vi "CSM Reuse Module.vi"(5 "Init State (\"Macro: Initialize\")":string="Macro: Initialize", 7 "Name (\"\" to Use UUID)":string="Reuse Module") -> ()   [LabVIEW 2017, in "1. Create a reuse Module.lvlib"]
doc: "#### Overview\n\nIn the CSM framework, creating a reusable module usually does not require message interaction with other modules. You only need to provide external interfaces and publish the module's state changes. Therefore, as long as these two aspects are clearly described, the reusable module can be called even without knowledge of its internal implementation details. This example demonstrates how to create a reusable module that checks if random data exceeds a user-defined threshold.\n\nIn a CSM module, all case branches can be considered callable messages, but it is recommended to use API groups as external interfaces. When state updates need to be sent, Status or Interrupt Status can be sent to notify external modules of internal state changes.\n\n#### Introduction\n\nThis example demonstrates a CSM module whose function is to generate a random number every second and compare that number with a user-defined threshold. When the generated random number exceeds the threshold, an update is broadcast.\n\n#### Steps\n\n- Step1: Drag and drop the CSM Template from the palette.\n- Step2: Add <b>Level</b> to Internal Data. The default value is 0.5.\n- Step3: Create \"DoSth: Check If Greater than 0.5\" to implement the core functionality.\n - Step3.1: Compare random data and update the UI.\n - Step3.2: Publish the \"Status Changed\" status when random data exceeds the level.\n- Step4: Change the <b>Timeout</b> to a shift register. It will be used to start/stop timeout events. Wire <b>Timeout</b> in every case.\n- Step5: In the Timeout Event, add \"DoSth: Check If Greater than 0.5\" to the State Queue.\n- Step6: Create APIs for this module.\n - Step6.1: Create \"API: Start\" to change the timeout to 0.5, which will trigger \"DoSth: Check If Greater than 0.5\" every second. In this case, broadcast the \"Check Started\" status.\n - Step6.2: Create \"API: Stop\" to change the timeout to -1, which will stop the checking. The \"Check Stopped\" status will be broadcast.\n - Step6.3: Create \"API: Set Level\" to change the Level setting.\n - Step6.4: Create \"API: Get Level\" to retrieve the current Level from the outside.\n- Step7: Create local test buttons/controls.\n - Step7.1: Create a <b>Level</b> control and call \"API: Set Level\" to change the level setting locally.\n - Step7.2: Create a <b>Start</b> button and call \"API: Start\" to begin checking locally.\n - Step7.3: Create a <b>Stop</b> button and call \"API: Stop\" to stop checking locally.\n- Step8: Correctly update the UI where appropriate.\n - Step8.1: Initialize the UI at startup.\n - Step8.2: Comment out `UI: Front Panel State >> Open` in \"Macro: Initialize\". When working as a submodule, the UI will automatically hide instead of popping up."
uses:
  1. Create a reuse Module.lvlib
  user.lib/_NEVSTOP/Communicable State Machine(CSM)/AdvanceAPI/CSM - Break Down Multiple States String.vi
  user.lib/_NEVSTOP/Communicable State Machine(CSM)/AdvanceAPI/CSM - Compact Multiple States.vi
  user.lib/_NEVSTOP/Communicable State Machine(CSM)/AdvanceAPI/CSM - Make String Arguments Safe.vi
  user.lib/_NEVSTOP/Communicable State Machine(CSM)/AdvanceAPI/CSM - Keywords.vi
  user.lib/_NEVSTOP/Communicable State Machine(CSM)/Communicable State Machine.lvlib
panel:
  in  "Level":dbl=0.5 min=0.0 max=1.0 step=0.1 format="%#_13g"
  in  "Stop":bool
  in  "Start":bool
  out "publish status":bool
  out "Random":dbl
  out "State History":string
  # "#CSM-Example Overview\n\nIn the CSM framework, creating a reusable module usually does not require message interaction with other modules. You only need to provide external interfaces and publish the module's state changes. Therefore, as long as these two aspects are clearly described, the reusable module can be called even without knowledge of its internal implementation details. This example demonstrates how to create a reusable module that checks if random data exceeds a user-defined threshold.\n\nIn a CSM module, all case branches can be considered callable messages, but it is recommended to use API groups as external interfaces. When state updates need to be sent, Status or Interrupt Status can be sent to notify external modules of internal state changes."
  # "If"
  # ">"
  # ", Then"
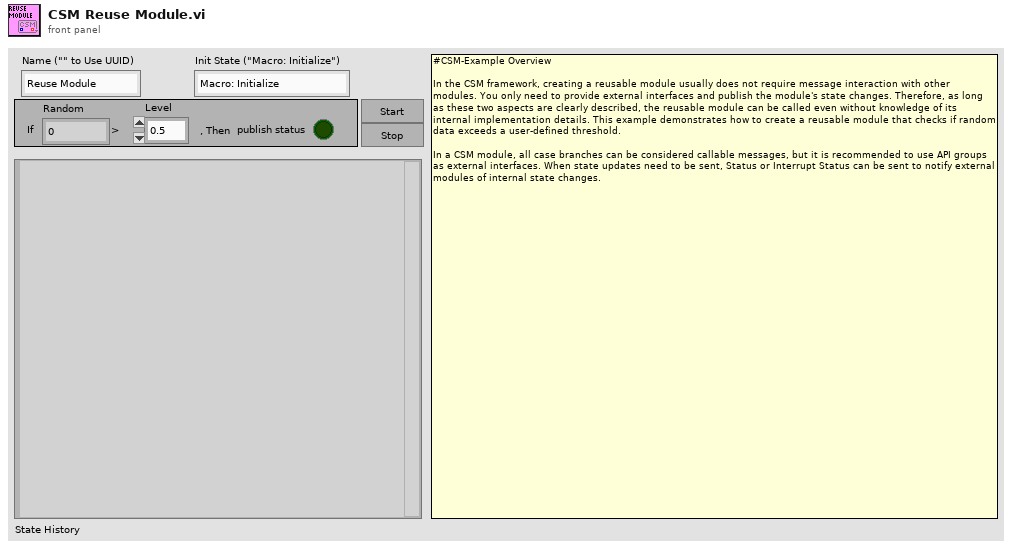
[diagram p1: front panel]
types:
  T1 = enum32{"Invalid", "Standard", "Closed", "Hidden", "Minimized", "Maximized"}
  T2 = enum32{"invalid app kind", "Development System", "Run Time System", "Student Edition", "Embedded LabVIEW", "Evaluation", "Custom"}
  T3 = typedef "Communicable State Machine.lvlib/_CSM_Response Source Message.ctl" = cluster{"‘State":string, "’Arguments":string, "’Error":errorcluster}
  T4 = cluster{"Current VI Reference":refnum<vi>, "Close Panel on Exit?":bool}
  T5 = cluster{"Core":cluster{"Current VI Reference":refnum<vi>, "Close Panel on Exit?":bool}, "Level":dbl}
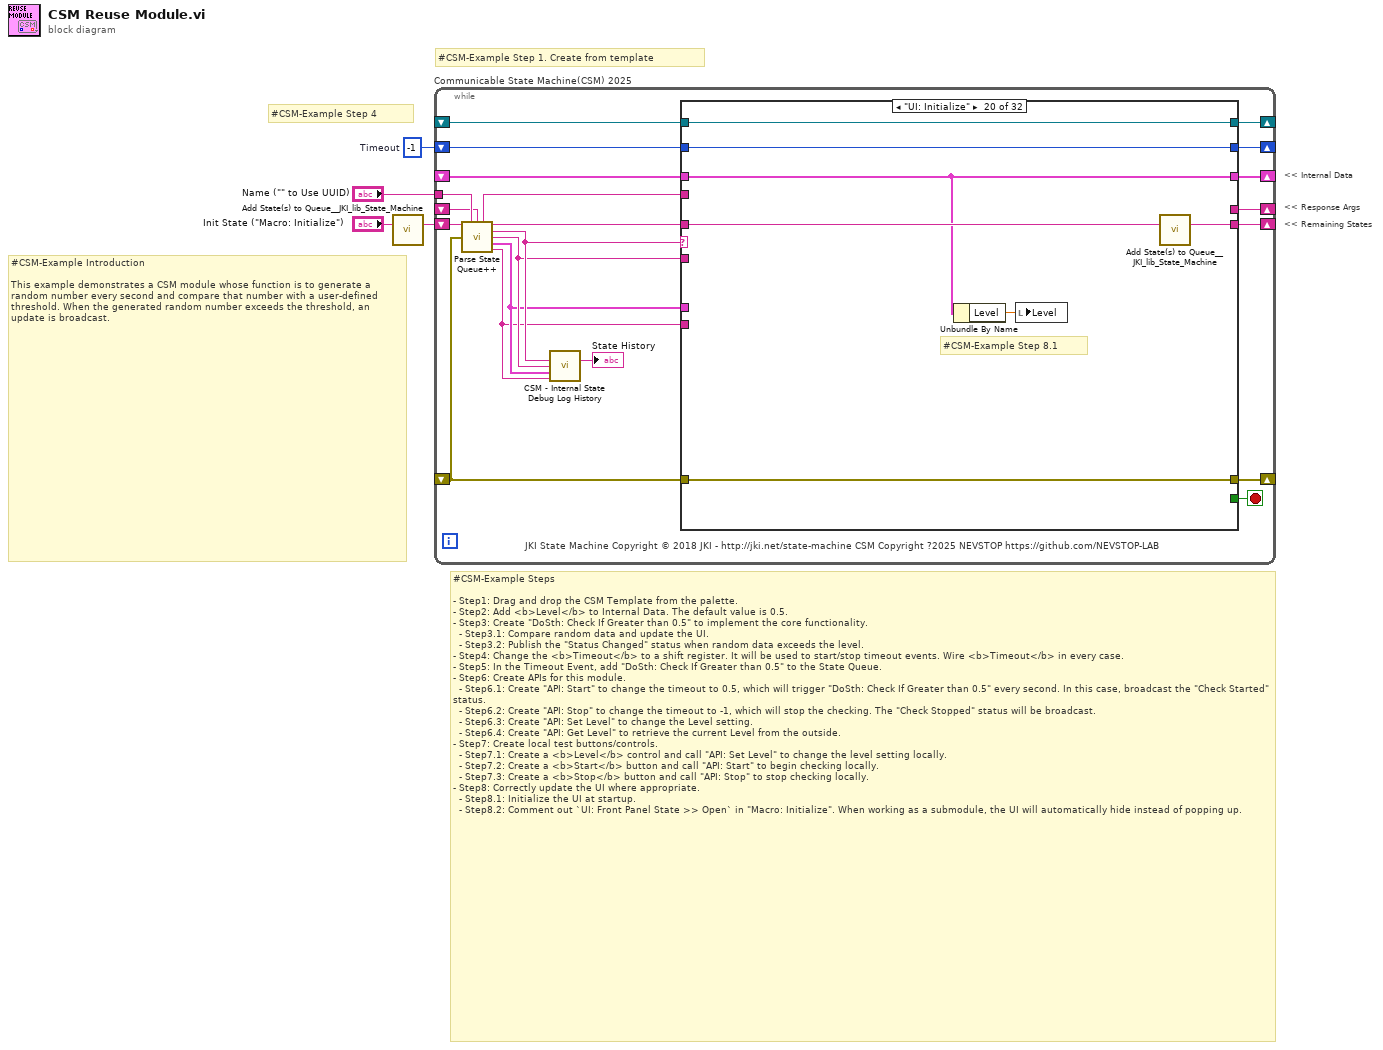
[diagram p0: block diagram]
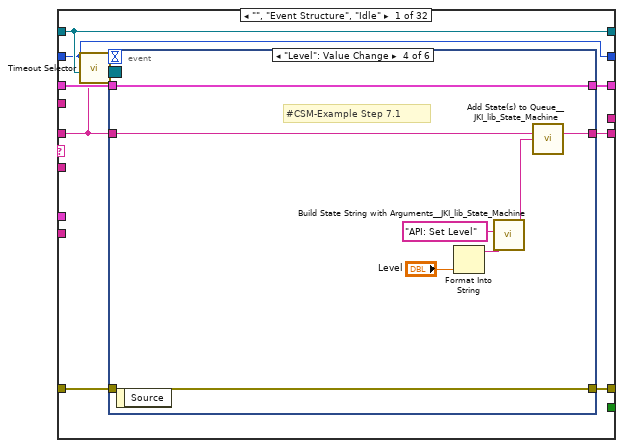
[diagram p2: hidden frame]
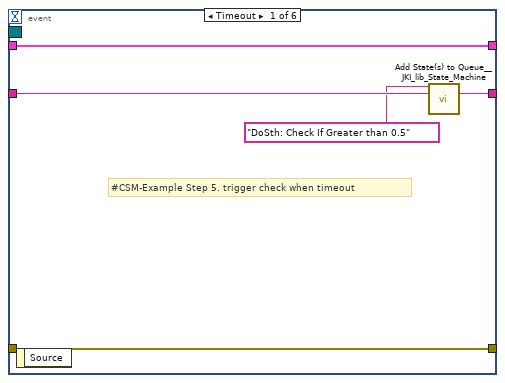
[diagram p3: hidden frame]
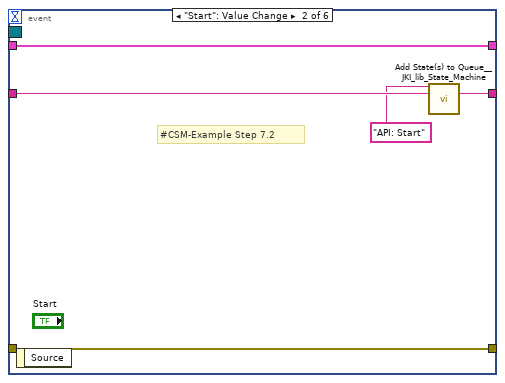
[diagram p4: hidden frame]
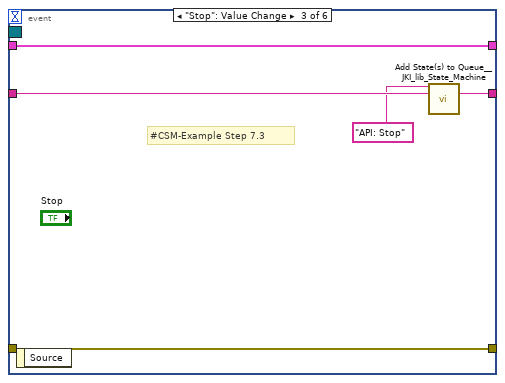
[diagram p5: hidden frame]
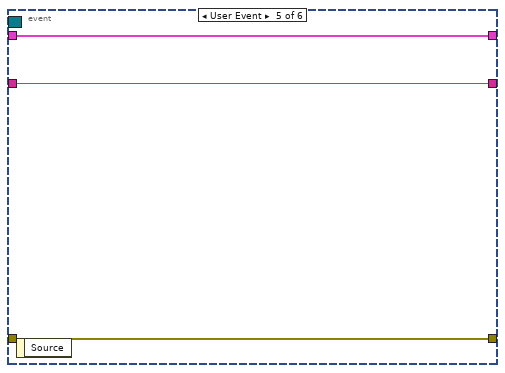
[diagram p6: hidden frame]
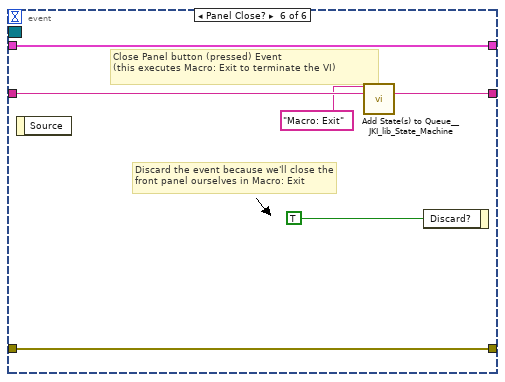
[diagram p7: hidden frame]
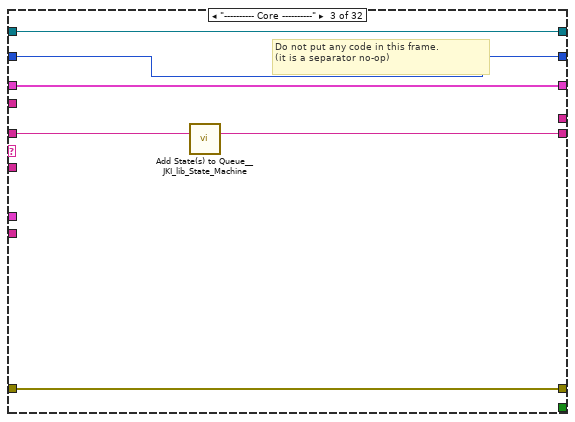
[diagram p9: hidden frame]
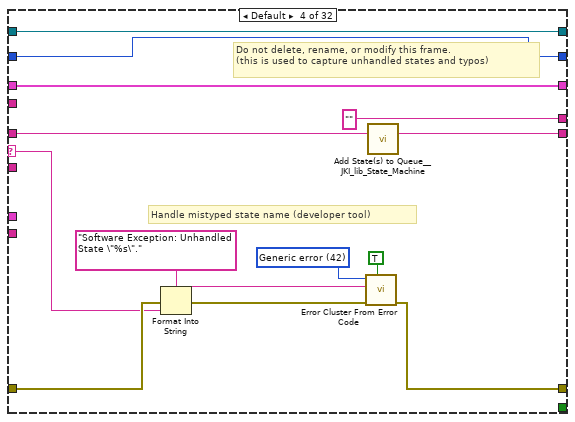
[diagram p10: hidden frame]
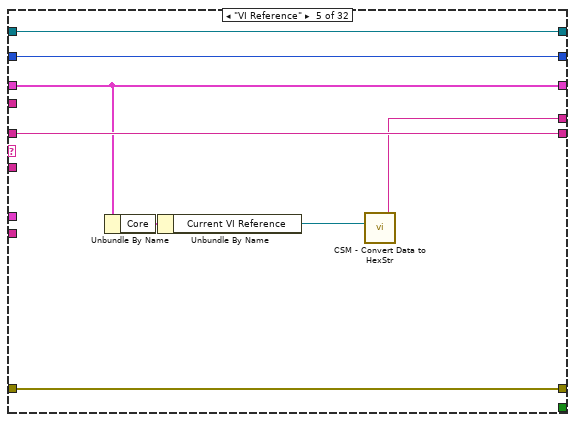
[diagram p11: hidden frame]
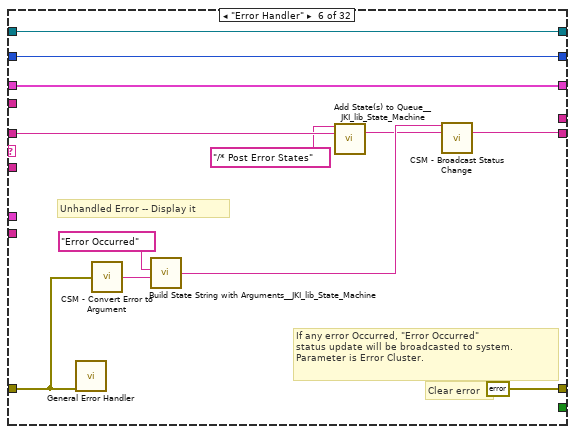
[diagram p12: hidden frame]
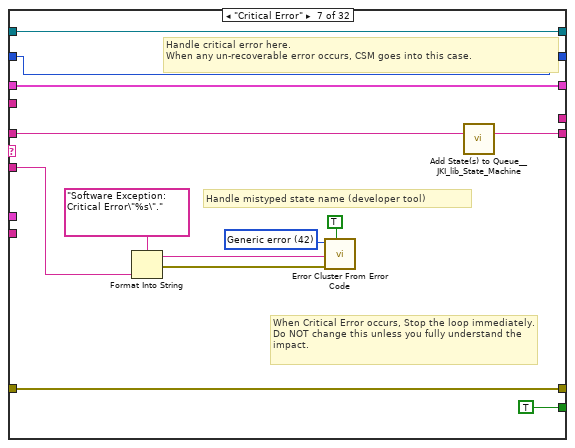
[diagram p13: hidden frame]
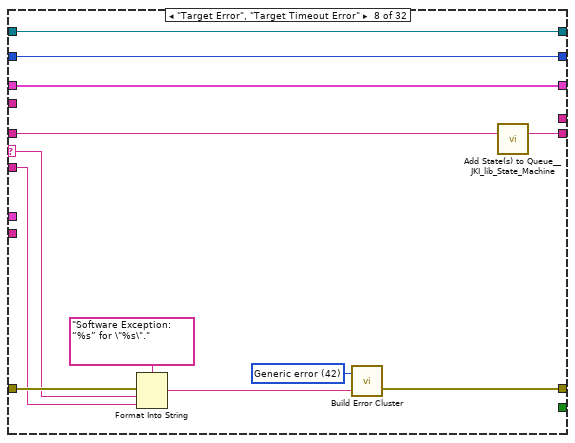
[diagram p14: hidden frame]
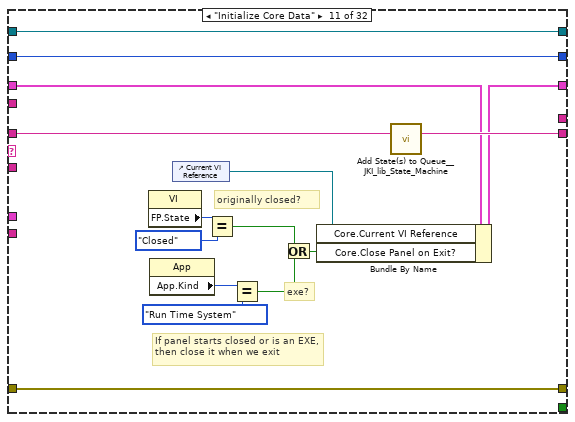
[diagram p17: hidden frame]
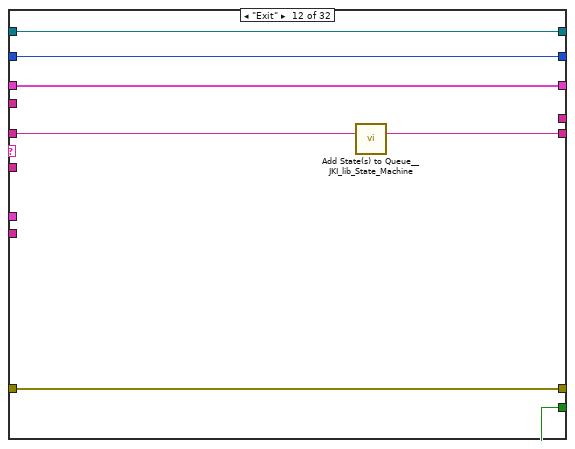
[diagram p18: hidden frame]
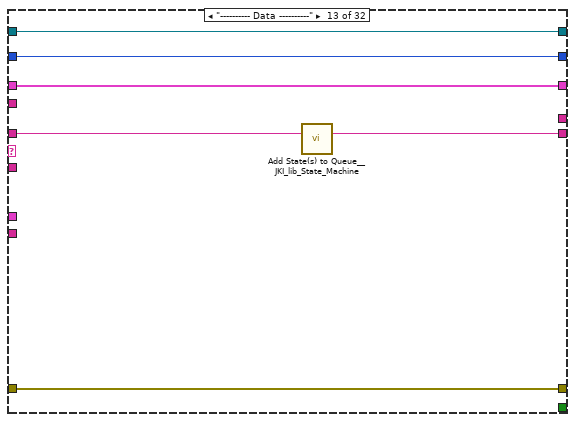
[diagram p19: hidden frame]
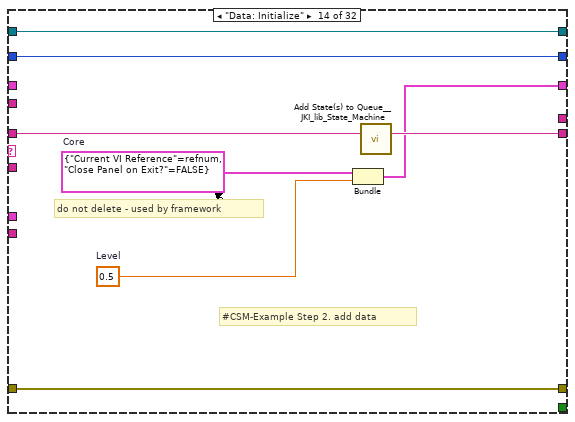
[diagram p20: hidden frame]
diagram:
  w2 = -1  # Timeout
  # "#CSM-Example Introduction\n\nThis example demonstrates a CSM module whose function is to generate a random number every second and compare that number with a user-defined threshold. When the generated random number exceeds the threshold, an update is broadcast."
  # "#CSM-Example Steps\n\n- Step1: Drag and drop the CSM Template from the palette.\n- Step2: Add <b>Level</b> to Internal Data. The default value is 0.5.\n- Step3: Create \"DoSth: Check If Greater than 0.5\" to implement the core functionality.\n  - Step3.1: Compare random data and update the UI.\n  - Step3.2: Publish the \"Status Changed\" status when random data exceeds the level.\n- Step4: Change the <b>Timeout</b> to a shift register. It will be used to start/stop timeout events. Wire <b>Timeout</b> in every case.\n- Step5: In the Timeout Event, add \"DoSth: Check If Greater than 0.5\" to the State Queue.\n- Step6: Create APIs for this module.\n  - Step6.1: Create \"API: Start\" to change the timeout to 0.5, which will trigger \"DoSth: Check If Greater than 0.5\" every second. In this case, broadcast the \"Check Started\" status.\n  - Step6.2: Create \"API: Stop\" to change the timeout to -1, which will stop the checking. The \"Check Stopped\" status will be broadcast.\n  - Step6.3: Create \"API: Set Level\" to change the Level setting.\n  - Step6.4: Create \"API: Get Level\" to retrieve the current Level from the outside.\n- Step7: Create local test buttons/controls.\n  - Step7.1: Create a <b>Level</b> control and call \"API: Set Level\" to change the level setting locally.\n  - Step7.2: Create a <b>Start</b> button and call \"API: Start\" to begin checking locally.\n  - Step7.3: Create a <b>Stop</b> button and call \"API: Stop\" to stop checking locally.\n- Step8: Correctly update the UI where appropriate.\n  - Step8.1: Initialize the UI at startup.\n  - Step8.2: Comment out `UI: Front Panel State >> Open` in \"Macro: Initialize\". When working as a submodule, the UI will automatically hide instead of popping up."
  # "#CSM-Example Step 4"
  # "#CSM-Example Step 1. Create from template"
  # "<< Internal Data"
  # "<< Response Args"
  # "<< Remaining States"
  n1 = call <vilib>:"Add State(s) to Queue__JKI_lib_State_Machine.vi"("State(s) in (\"\")"="Init State (\"Macro: Initialize\")") -> ("States Out"=w4:string)  [unwired: 14 in]
  n2 = while "Communicable State Machine(CSM) 2025" {
    shift-right: [w20] -> _
    shift-left: _ -> [w19]
    shift-right: [w23] -> _
    shift-left: _ -> [w18]
    shift-right: [w22] -> _
    shift-left: w4 -> [w24]
    tunnel: "Name (\"\" to Use UUID)" -> [w14]
    shift-right: [w17] -> _
    shift-left: _ -> [w8]
    shift-right: [w16] -> _
    shift-left: _ -> [w15]
    shift-right: [w6] -> _
    shift-left: w2 -> [w7]
    stop <- w21 stop-if-true
    # "JKI State Machine Copyright © 2018 JKI - http://jki.net/state-machine CSM Copyright ?2025 NEVSTOP https://github.com/NEVSTOP-LAB"
    n3 = call "Parse State Queue++.vi"("State Queue"=w24, "Name (\"\" to Use UUID)"=w14, "Response Arguments"=w8, "Previous Error"=w18) -> ("Name Used"=w9:string, "Remaining States"=w25:string, "Current State"=w13:string, "Arguments"=w12:string, "Additional Information"=w11:T3, "Source CSM"=w10:string)  [unwired: 6 in]
    n4 = call "CSM - Internal State Debug Log History.vi"("State"=w13, "Arguments (\"\")"=w12, ">> Response Source Message >>"=w11, "Source (\"\")"=w10) -> ("Debug Log"=→"State History":string)  [unwired: 11 in]
    n5 = case shown="\"UI: Initialize\"" w13 {
      selector: w13 -> [_ _ _ w81 _ _ _ w126 _ _ _ _ _ _ _ _ _ _ _ _ _ _ _ _ _ _ _ _ _ _ _ _]
      tunnel: w25 -> [w27 w70 w77 w85 w98 w111 w122 w128 w140 w145 w161 w168 w174 w182 w190 w196 w203 w208 w215 w222 w230 w247 w318 w325 w337 w341 w348 w355 w363 w370 w377 w391]
      tunnel: w12 -> [_ _ _ _ _ _ w115 w127 _ _ _ _ _ _ _ _ _ _ _ _ w225 w241 _ _ _ _ _ _ w358 _ _ _]
      tunnel: w19 -> [w33 w69 w74 w83 w97 w109 w123 w130 w139 w144 w154 w166 w171 _ w185 w193 w202 w207 w212 w217 w228 w243 w315 w322 w334 w340 w347 w354 w362 w367 w374 w382]
      tunnel: [w32 w71 w75 w87 w99 errorcluster {"status"=FALSE, "code"=0, "source"=""} ("error out") w124 w133 w141 w146 w158 w165 w172 w179 w186 w194 w198 w206 w213 w220 w226 w244 w316 w323 w335 w342 w349 w356 w364 w371 w375 w389] -> w23
      tunnel: w18 -> [w31 w71 w75 w86 w99 w100 w124 w132 w141 w146 w158 w165 w172 w179 w187 w194 _ w209 w213 w220 w227 w245 w316 w323 w335 w342 w349 w356 w364 w371 w375 w389]
      tunnel: [w34 w70 w76 w84 w98 w102 w121 w131 w140 w145 w160 w167 w173 w181 w189 w195 w203 w208 w214 w221 w229 w246 w317 w324 w336 w341 w344 w351 w363 w370 w376 w390] -> w22
      tunnel: [_ _ _ _ _ _ TRUE _ _ _ _ TRUE _ _ _ _ _ _ _ _ _ _ _ _ _ _ _ _ _ _ _ _] -> w21
      tunnel: [w30 w69 w74 w83 w97 w109 w123 w130 w139 w144 w159 w166 w171 w180 w185 w193 w202 w207 w212 w217 w228 w243 w315 w322 w334 w340 w347 w354 w359 w367 w374 w382] -> w20
      tunnel: w7 -> [w26 w67 w72 w78 w95 w101 w112 w125 w137 w142 w147 w162 w169 w176 w183 w191 w197 w204 w210 w218 w223 w239 w313 w319 w326 w338 _ _ w360 w368 w372 w383]
      tunnel: w10 -> [_ _ _ _ _ _ _ _ _ _ _ _ _ _ _ _ _ _ _ _ _ _ _ _ _ _ _ _ _ _ _ _]
      tunnel: w11 -> [_ _ _ _ _ _ _ _ _ _ _ _ _ _ _ _ _ _ _ _ _ _ _ _ _ _ _ _ _ _ _ _]
      tunnel: [_ _ _ "" w92 _ _ _ _ _ _ _ _ _ _ _ _ _ _ _ _ _ _ _ _ _ _ _ _ w365 _ _] -> w17
      tunnel: [w29 w68 w73 w79 w96 w107 w113 w129 w138 w143 w148 w163 w170 w177 w184 w192 w201 w205 w211 w219 w224 w240 w314 w320 w327 w339 w346 w353 w361 w369 w373 w388] -> w16
      tunnel: w15 -> [w29 w68 w73 w79 w96 w107 w113 w129 w138 w143 w148 w163 w170 w177 w184 w192 _ w205 w211 w219 w224 w240 w314 w320 w327 w339 w346 w353 w361 w369 w373 w388]
      tunnel: w9 -> [_ _ _ _ _ _ _ _ _ _ _ _ _ _ _ _ w200 _ _ _ _ _ _ _ _ _ _ _ _ _ _ _]
      tunnel: [w26 w67 w72 w78 w95 w101 w112 w125 w137 w142 w147 w162 w169 w176 w183 w191 w197 w204 w210 w218 w223 w239 w313 w319 w326 w338 500 ("Timeout") -1 ("Timeout") w360 w368 w372 w383] -> w6
      frame "", "Event Structure", "Idle" {
        n6 = call "Timeout Selector.vi"("Remaining States"=w27, "Timeout Expected"=w26) -> ("Timeout"=w28:i32)  [unwired: 5 in]
        n7 = event shown="[3] \"Level\": Value Change" {
          selector: w29 -> [_ _ _ _ _ _]
          dyn-events: _ -> [_ _ _ _ _ _]
          timeout: w28 -> [_ _ _ _ _ _]
          tunnel: w27 -> [w39 w44 w49 w55 w59 w66]
          tunnel: [w38 w43 w48 w54 w59 w65] -> w34
          tunnel: w33 -> [w36 w41 w46 w56 w60 w63]
          tunnel: [w37 w42 w47 w57 w58 w64] -> w32
          tunnel: w31 -> [w37 w42 w47 w57 w58 w64]
          tunnel: [w36 w41 w46 w56 w60 w63] -> w30
          event Timeout {
            # "#CSM-Example Step 5. trigger check when timeout"
            n8 = event-data() -> ()  [unwired: 1 in, 1 out]
            n9 = call <vilib>:"Add State(s) to Queue__JKI_lib_State_Machine.vi"("State(s) in Front (\"\")"="DoSth: Check If Greater than 0.5" ("State(s) in Front (\"\")"), "State(s) in (\"\")"=w39) -> ("States Out"=w38:string)  [unwired: 13 in]
          }
          event "Start": Value Change {
            # "#CSM-Example Step 7.2"
            n10 = event-data() -> ()  [unwired: 1 in, 1 out]
            n11 = call <vilib>:"Add State(s) to Queue__JKI_lib_State_Machine.vi"("State(s) in Front (\"\")"="API: Start" ("State(s) in Front (\"\")"), "State(s) in (\"\")"=w44) -> ("States Out"=w43:string)  [unwired: 13 in]
          }
          event "Stop": Value Change {
            # "#CSM-Example Step 7.3"
            n12 = event-data() -> ()  [unwired: 1 in, 1 out]
            n13 = call <vilib>:"Add State(s) to Queue__JKI_lib_State_Machine.vi"("State(s) in Front (\"\")"="API: Stop" ("State(s) in Front (\"\")"), "State(s) in (\"\")"=w49) -> ("States Out"=w48:string)  [unwired: 13 in]
          }
          event "Level": Value Change {
            # "#CSM-Example Step 7.1"
            n14 = event-data() -> ()  [unwired: 1 in, 1 out]
            n15 = Format Into String("Level") -> (resulting string=w50:string)  [unwired: 3 in, 1 out]
            n16 = call <vilib>:"Build State String with Arguments__JKI_lib_State_Machine.vi"("Arguments (\"\")"=w50, "State"="API: Set Level") -> ("State with Arguments"=w53:string)  [unwired: 4 in]
            n17 = call <vilib>:"Add State(s) to Queue__JKI_lib_State_Machine.vi"("State(s) in (\"\")"=w55, "State(s) at Back (\"\")"=w53) -> ("States Out"=w54:string)  [unwired: 13 in]
          }
          event User Event {
            n18 = event-data() -> ()  [unwired: 1 in, 1 out]
          }
          event Panel Close? {
            # "Discard the event because we'll close the front panel ourselves in Macro: Exit"
            # "Close Panel button (pressed) Event\n(this executes Macro: Exit to terminate the VI)"
            n19 = event-data() -> ()  [unwired: 1 in, 1 out]
            n20 = call <vilib>:"Add State(s) to Queue__JKI_lib_State_Machine.vi"("State(s) in Front (\"\")"="Macro: Exit", "State(s) in (\"\")"=w66) -> ("States Out"=w65:string)  [unwired: 13 in]
            n21 = event-data("Discard?"=TRUE) -> ()  [unwired: 1 in, 1 out]
          }
        }
      }
      frame "CSM Documentation" {
        # "#CSM README FIRST\n\nCSM is a LabVIEW application framework that builds upon JKI State Machine (JKISM). It follows the pattern of JKISM and extends the keywords to describe message communication between CSM modules, including concepts such as Sync-Message, Async-Message, Subscription/Unsubscription of status - essential elements for creating reusable code modules. For more information, please visit the CSM wiki: https://github.com/NEVSTOP-LAB/JKI-State-Machine-Plus-Plus/wiki\n\nFor instructions on JKI State Machine, visit: http://jki.net/state-machine/\nFor information about CSM, visit: https://github.com/NEVSTOP-LAB"
        # "CSM Documentation"
      }
      frame "---------- Core ----------" {
        # "Do not put any code in this frame.\n(it is a separator no-op)"
        n22 = call <vilib>:"Add State(s) to Queue__JKI_lib_State_Machine.vi"("State(s) in (\"\")"=w77) -> ("States Out"=w76:string)  [unwired: 14 in]
      }
      frame Default {
        w90 = 42 items=["No error", "Argument error", "Memory is full", "Out of zone", "End of file", "File already open", "Generic file I/O error", "File not found", "File permission error", "Disk is full", "Duplicate path", "Too many files open", "System feature not enabled", "Resource file not found", "Cannot add resource", "Resource not found", "Image not found", "Image memory error", "Pen does not exist", "Config type invalid", "Config token not found", "Config parse error", "Config memory error", "Bad external code format", "Bad external code offset", "External code not present", "Null window", "Destroy window error", "Null menu", "Print aborted", "Bad print record", "Print driver error", "Windows error during printing", "Memory error during printing", "Print dialog error", "Generic print error", "Invalid device refnum", "Device not found", "Device parameter error", "Device unit error", "Cannot open device", "Device call aborted", "Generic error", "Cancelled by user", "Object ID too low", "Object ID too high", "Object not in heap", "Unknown heap", "Unknown object (invalid DefProc)", "Unknown object (DefProc not in table)", "Message out of range", "Invalid (null) method", "Unknown message", "Manager call not supported", "Bad address", "Network operation in progress", "Network operation timed out", "Connection is busy", "Network attribute not supported", "Network error", "Address in use", "System out of memory", "Connection aborted", "Connection refused", "Not connected", "Already connected", "Connection closed", "Initialization error (interapplication manager)", "Bad occurrence", "Wait on unbound occurrence handler", "Occurrence queue overflow", "Datalog type conflict", "Unused", "Unrecognized type (interapplication manager)", "Memory corrupt", "Failed to make temporary DLL", "Old CIN version", "Drag socket not found", "Failed to load drop-object", "Failed to register OLE object", "Failed to release OLE object", "Format specifier type mismatch", "Unknown format specifier", "Too few format specifiers", "Too many format specifiers", "Scan failed", "Newer CIN version", "Error converting to variant", "Runtime menu error", "Password tampered", "Variant attribute not found", "Incompatible variant data type", "Event data is not available", "Event Store is not present", "Occurrence is not found", "Event Queue is not created", "Event info is not available", "Refnum passed is NULL", "Error retrieving Class GUID", "Error retrieving CoClass GUID", "Error retrieving TypeLib GUID.", "Bad built application magic bytes.", "Specific driver is different from the specific driver associated with the Logical Name.", "There is no session opened to the class driver.", "Max Error", "MAX - Error with config objects", "MAX - Error loading configuration", "MAX - Group not supported"]
        # "Do not delete, rename, or modify this frame.\n(this is used to capture unhandled states and typos)"
        # "Handle mistyped state name (developer tool)"
        n23 = Format Into String(format string="Software Exception: Unhandled State \"%s\"." ("message"), error in=w86, w81) -> (resulting string=w89:string, error out=w88:errorcluster)  [unwired: 1 in]
        n24 = call <vilib>:"Error Cluster From Error Code.vi"("show call chain? (False)"=TRUE, "error in (no error)"=w88, "error message (\"\")"=w89, "error code (0)"=w90) -> ("error out"=w87:errorcluster)  [unwired: 5 in]
        n25 = call <vilib>:"Add State(s) to Queue__JKI_lib_State_Machine.vi"("State(s) in (\"\")"=w85) -> ("States Out"=w84:string)  [unwired: 14 in]
      }
      frame "VI Reference" {
        n26 = Unbundle By Name(w97) -> ("Core"=w94:T4)
        n27 = Unbundle By Name(w94) -> ("Current VI Reference"=w93:refnum<vi>)
        n28 = call "CSM - Convert Data to HexStr.vi"("Variant"=w93) -> ("HEX String (0-9,A-F)"=w92:string)  [unwired: 8 in]
      }
      frame "Error Handler" {
        # "If any error Occurred, \"Error Occurred\" \nstatus update will be broadcasted to system.\nParameter is Error Cluster."
        # "Unhandled Error -- Display it"
        # "Clear error"
        n29 = call <vilib>:"General Error Handler.vi"("error in (no error)"=w100) -> ()  [unwired: 10 in, 5 out]
        n30 = call "CSM - Convert Error to Argument.vi"("Error"=w100) -> ("Argument"=w105:string)  [unwired: 4 in]
        n31 = call <vilib>:"Build State String with Arguments__JKI_lib_State_Machine.vi"("Arguments (\"\")"=w105, "State"="Error Occurred" ("Status with Arguments")) -> ("State with Arguments"=w104:string)  [unwired: 4 in]
        n32 = call <vilib>:"Add State(s) to Queue__JKI_lib_State_Machine.vi"("State(s) in Front (\"\")"="/* Post Error States", "State(s) in (\"\")"=w111) -> ("States Out"=w103:string)  [unwired: 13 in]
        n33 = call "CSM - Broadcast Status Change.vi"("Status With Arguments"=w104, "State Queue"=w103) -> ("Remaining States"=w102:string)  [unwired: 13 in]
      }
      frame "Critical Error" {
        w119 = 42 items=["No error", "Argument error", "Memory is full", "Out of zone", "End of file", "File already open", "Generic file I/O error", "File not found", "File permission error", "Disk is full", "Duplicate path", "Too many files open", "System feature not enabled", "Resource file not found", "Cannot add resource", "Resource not found", "Image not found", "Image memory error", "Pen does not exist", "Config type invalid", "Config token not found", "Config parse error", "Config memory error", "Bad external code format", "Bad external code offset", "External code not present", "Null window", "Destroy window error", "Null menu", "Print aborted", "Bad print record", "Print driver error", "Windows error during printing", "Memory error during printing", "Print dialog error", "Generic print error", "Invalid device refnum", "Device not found", "Device parameter error", "Device unit error", "Cannot open device", "Device call aborted", "Generic error", "Cancelled by user", "Object ID too low", "Object ID too high", "Object not in heap", "Unknown heap", "Unknown object (invalid DefProc)", "Unknown object (DefProc not in table)", "Message out of range", "Invalid (null) method", "Unknown message", "Manager call not supported", "Bad address", "Network operation in progress", "Network operation timed out", "Connection is busy", "Network attribute not supported", "Network error", "Address in use", "System out of memory", "Connection aborted", "Connection refused", "Not connected", "Already connected", "Connection closed", "Initialization error (interapplication manager)", "Bad occurrence", "Wait on unbound occurrence handler", "Occurrence queue overflow", "Datalog type conflict", "Unused", "Unrecognized type (interapplication manager)", "Memory corrupt", "Failed to make temporary DLL", "Old CIN version", "Drag socket not found", "Failed to load drop-object", "Failed to register OLE object", "Failed to release OLE object", "Format specifier type mismatch", "Unknown format specifier", "Too few format specifiers", "Too many format specifiers", "Scan failed", "Newer CIN version", "Error converting to variant", "Runtime menu error", "Password tampered", "Variant attribute not found", "Incompatible variant data type", "Event data is not available", "Event Store is not present", "Occurrence is not found", "Event Queue is not created", "Event info is not available", "Refnum passed is NULL", "Error retrieving Class GUID", "Error retrieving CoClass GUID", "Error retrieving TypeLib GUID.", "Bad built application magic bytes.", "Specific driver is different from the specific driver associated with the Logical Name.", "There is no session opened to the class driver.", "Max Error", "MAX - Error with config objects", "MAX - Error loading configuration", "MAX - Group not supported"]
        # "Handle critical error here.\nWhen any un-recoverable error occurs, CSM goes into this case."
        # "When Critical Error occurs, Stop the loop immediately. Do NOT change this unless you fully understand the impact."
        # "Handle mistyped state name (developer tool)"
        n34 = Format Into String(format string="Software Exception: Critical Error\"%s\"." ("message"), w115) -> (resulting string=w118:string, error out=w117:errorcluster)  [unwired: 2 in]
        n35 = call <vilib>:"Error Cluster From Error Code.vi"("show call chain? (False)"=TRUE, "error in (no error)"=w117, "error message (\"\")"=w118, "error code (0)"=w119) -> ()  [unwired: 5 in, 1 out]
        n36 = call <vilib>:"Add State(s) to Queue__JKI_lib_State_Machine.vi"("State(s) in (\"\")"=w122) -> ("States Out"=w121:string)  [unwired: 14 in]
      }
      frame "Target Error", "Target Timeout Error" {
        w135 = 42 items=["No error", "Argument error", "Memory is full", "Out of zone", "End of file", "File already open", "Generic file I/O error", "File not found", "File permission error", "Disk is full", "Duplicate path", "Too many files open", "System feature not enabled", "Resource file not found", "Cannot add resource", "Resource not found", "Image not found", "Image memory error", "Pen does not exist", "Config type invalid", "Config token not found", "Config parse error", "Config memory error", "Bad external code format", "Bad external code offset", "External code not present", "Null window", "Destroy window error", "Null menu", "Print aborted", "Bad print record", "Print driver error", "Windows error during printing", "Memory error during printing", "Print dialog error", "Generic print error", "Invalid device refnum", "Device not found", "Device parameter error", "Device unit error", "Cannot open device", "Device call aborted", "Generic error", "Cancelled by user", "Object ID too low", "Object ID too high", "Object not in heap", "Unknown heap", "Unknown object (invalid DefProc)", "Unknown object (DefProc not in table)", "Message out of range", "Invalid (null) method", "Unknown message", "Manager call not supported", "Bad address", "Network operation in progress", "Network operation timed out", "Connection is busy", "Network attribute not supported", "Network error", "Address in use", "System out of memory", "Connection aborted", "Connection refused", "Not connected", "Already connected", "Connection closed", "Initialization error (interapplication manager)", "Bad occurrence", "Wait on unbound occurrence handler", "Occurrence queue overflow", "Datalog type conflict", "Unused", "Unrecognized type (interapplication manager)", "Memory corrupt", "Failed to make temporary DLL", "Old CIN version", "Drag socket not found", "Failed to load drop-object", "Failed to register OLE object", "Failed to release OLE object", "Format specifier type mismatch", "Unknown format specifier", "Too few format specifiers", "Too many format specifiers", "Scan failed", "Newer CIN version", "Error converting to variant", "Runtime menu error", "Password tampered", "Variant attribute not found", "Incompatible variant data type", "Event data is not available", "Event Store is not present", "Occurrence is not found", "Event Queue is not created", "Event info is not available", "Refnum passed is NULL", "Error retrieving Class GUID", "Error retrieving CoClass GUID", "Error retrieving TypeLib GUID.", "Bad built application magic bytes.", "Specific driver is different from the specific driver associated with the Logical Name.", "There is no session opened to the class driver.", "Max Error", "MAX - Error with config objects", "MAX - Error loading configuration", "MAX - Group not supported"]
        n37 = Format Into String(format string="Software Exception: “%s” for \"%s\"." ("message"), error in=w132, w126, w127) -> (resulting string=w134:string)  [unwired: 1 in, 1 out]
        n38 = call "Build Error Cluster.vi"("String to Prepend to Source (\"\")"=w134, "Code"=w135) -> ("error out"=w133:errorcluster)
        n39 = call <vilib>:"Add State(s) to Queue__JKI_lib_State_Machine.vi"("State(s) in (\"\")"=w128) -> ("States Out"=w131:string)  [unwired: 14 in]
      }
      frame "Async Response", "Response" {
        # "Handle Async-call Response (\"Async Response\" for ->)"
        # "Handle Sync-call Response (\"Response\" for @)"
        # "After Message is executed, CSM goes to this state for receive the response. \n    For Async Message(->), \"Async Response\" is used. This CSM will goes to \"Async Message Posted\" immediately and receive the \"Async Response\" after the callee finishes the message.\n    For Sync Message(@),  This CSM will wait until the message is done and immediately goes to \"Response\""
      }
      frame "Async Message Posted" {
        # "Handle post action for async message (->)."
        # "After Async Message is posted (->), CSM goes to this state for post-action. You can use Argument - State to tell which Async Message is called."
      }
      frame "Initialize Core Data" {
        # "originally closed?"
        # "exe?"
        # "If panel starts closed or is an EXE, then close it when we exit"
        n40 = property class="VI"() -> ("FP.State"=w151:T1)  [unwired: 2 in, 2 out]
        n41 = property class="App"() -> ("App.Kind"=w157:T2)  [unwired: 2 in, 2 out]
        n42 = control-ref of="Current VI Reference"() -> (w152:refnum<vi>)
        n43 = Equal?(x=w151, y=T1."Closed" ("Front Panel Window:State")) -> (x = y?=w149:bool)
        n44 = Equal?(x=w157, y=T2."Run Time System" ("Application:Kind")) -> (x = y?=w155:bool)
        n45 = Or(x=w149, y=w155) -> (x .or. y?=w153:bool)
        n46 = Bundle By Name(cluster=w154, "Core.Current VI Reference"=w152, "Core.Close Panel on Exit?"=w153) -> (w159:T5)
        n47 = call <vilib>:"Add State(s) to Queue__JKI_lib_State_Machine.vi"("State(s) in (\"\")"=w161) -> ("States Out"=w160:string)  [unwired: 14 in]
      }
      frame "Exit" {
        n48 = call <vilib>:"Add State(s) to Queue__JKI_lib_State_Machine.vi"("State(s) in (\"\")"=w168) -> ("States Out"=w167:string)  [unwired: 14 in]
      }
      frame "---------- Data ----------" {
        n49 = call <vilib>:"Add State(s) to Queue__JKI_lib_State_Machine.vi"("State(s) in (\"\")"=w174) -> ("States Out"=w173:string)  [unwired: 14 in]
      }
      frame "Data: Initialize" {
        w175 = 0.5  # Level
        w178 = T4 {"Current VI Reference"=refnum, "Close Panel on Exit?"=FALSE}  # Core
        # "#CSM-Example Step 2. add data"
        # "do not delete - used by framework"
        n50 = Bundle("Core"=w178, "Level"=w175) -> (w180:T5)  [unwired: 1 in]
        n51 = call <vilib>:"Add State(s) to Queue__JKI_lib_State_Machine.vi"("State(s) in (\"\")"=w182) -> ("States Out"=w181:string)  [unwired: 14 in]
      }
      frame "Data: Cleanup" {
        n52 = Unbundle By Name(w185) -> ("Core.Current VI Reference"=w188:refnum<vi>)
        n53 = Close Reference(reference=w188, error in (no error)=w187) -> (error out=w186:errorcluster)
        n54 = call <vilib>:"Add State(s) to Queue__JKI_lib_State_Machine.vi"("State(s) in (\"\")"=w190) -> ("States Out"=w189:string)  [unwired: 14 in]
      }
      frame "---------- Events ----------" {
        n55 = call <vilib>:"Add State(s) to Queue__JKI_lib_State_Machine.vi"("State(s) in (\"\")"=w196) -> ("States Out"=w195:string)  [unwired: 14 in]
      }
      frame "Events: Register" {
        # "Register message event to break Waiting in Event structure."
        n56 = call "CSM - Get New State Notifier Event.vi"("Name (\"\" to Use UUID)"=w200) -> ("error out"=w198:errorcluster, "New State Notifier Event"=w199:refnum<user-event>)  [unwired: 9 in]
        n57 = register-events(w199) -> (reference out=w201:refnum<event-registration>)  [unwired: 2 in, 1 out]
      }
      frame "Events: Unregister" {
        n58 = Unregister For Events(event registration refnum=w205, error in=w209) -> (error out=w206:errorcluster)
      }
      frame "---------- UI ----------" {
        n59 = call <vilib>:"Add State(s) to Queue__JKI_lib_State_Machine.vi"("State(s) in (\"\")"=w215) -> ("States Out"=w214:string)  [unwired: 14 in]
      }
      frame "UI: Initialize" {
        # "#CSM-Example Step 8.1"
        n60 = Unbundle By Name(w217) -> ("Level"=w216:dbl)
        n61 = local write "Level"(w216) -> ()
        n62 = call <vilib>:"Add State(s) to Queue__JKI_lib_State_Machine.vi"("State(s) in (\"\")"=w222) -> ("States Out"=w221:string)  [unwired: 14 in]
      }
      frame "UI: Cursor Set" {
        # "Argument"
        n63 = disable-structure shown="TARGET_TYPE!=Windows" {
          disable-tunnel: w227 -> [w233 w238]
          disable-tunnel: [w232 w238] -> w226
          disable-tunnel: w225 -> [w231 _]
          frame condition #0 (active) {
            n64 = case shown="\"Idle\", Default" w231 {
              tunnel: w233 -> [w235 w237]
              tunnel: [w234 w236] -> w232
              frame "Idle", Default {
                n65 = call <vilib>:"Unset Busy.vi"("error in (no error)"=w235) -> ("error out"=w234:errorcluster)  [unwired: 10 in]
              }
              frame "Busy" {
                n66 = call <vilib>:"Set Busy.vi"("error in (no error)"=w237) -> ("error out"=w236:errorcluster)  [unwired: 9 in, 1 out]
              }
            }
          }
          frame condition #1 {
          }
        }
        n67 = call <vilib>:"Add State(s) to Queue__JKI_lib_State_Machine.vi"("State(s) in (\"\")"=w230) -> ("States Out"=w229:string)  [unwired: 14 in]
      }
      frame "UI: Front Panel State" {
        # "Argument"
        n68 = Unbundle By Name(w243) -> ("Core.Current VI Reference"=w242:refnum<vi>)
        n69 = call <vilib>:"Add State(s) to Queue__JKI_lib_State_Machine.vi"("State(s) in (\"\")"=w247) -> ("States Out"=w246:string)  [unwired: 14 in]
        n70 = case shown="\"Close\", \"Closed\"" w241 {
          tunnel: w245 -> [w253 w268 w279 w292 w305]
          tunnel: [w255 w269 w281 w294 w307] -> w244
          tunnel: w242 -> [w254 w266 w280 w293 w306]
          frame "Open", "Standard", Default {
            w248 = T1."Standard" ("State")
            n71 = property class="VI"(reference=w254, error in=w253) -> (reference out=w251:refnum<vi>, error out=w252:errorcluster, "FP.State"=w250:T1)
            n72 = Not Equal?(x=w250, y=w248) -> (x != y?=w249:bool)
            n73 = case shown="True" w249 {
              tunnel: [w259 w261] -> w255
              tunnel: w252 -> [w258 w261]
              tunnel: w251 -> [w257 _]
              tunnel: w248 -> [w256 _]
              frame True {
                n74 = invoke class="VI" method="FP.Open"(reference=w257, error in=w258, "Activate"=TRUE, "State"=w256) -> (error out=w259:errorcluster)  [unwired: 1 in, 4 out]
              }
              frame False {
              }
            }
          }
          frame "Close", "Closed" {
            n75 = property class="VI"(reference=w266, error in=w268) -> (reference out=w265:refnum<vi>, error out=w267:errorcluster, "FP.State"=w263:T1)
            n76 = Not Equal?(x=w263, y=T1."Closed" ("Front Panel Window:State")) -> (x != y?=w262:bool)
            n77 = case shown="True" w262 {
              tunnel: [w270 w273] -> w269
              tunnel: w267 -> [w270 w272]
              tunnel: w265 -> [_ w271]
              frame False {
              }
              frame True {
                n78 = invoke class="VI" method="FP.Close"(reference=w271, error in=w272) -> (error out=w273:errorcluster)  [unwired: 1 in, 2 out]
              }
            }
          }
          frame "Hidden", "Hide" {
            w274 = T1."Hidden" ("State")
            n79 = property class="VI"(reference=w280, error in=w279) -> (reference out=w277:refnum<vi>, error out=w278:errorcluster, "FP.State"=w276:T1)
            n80 = Not Equal?(x=w276, y=w274) -> (x != y?=w275:bool)
            n81 = case shown="True" w275 {
              tunnel: [w285 w286] -> w281
              tunnel: w278 -> [w284 w286]
              tunnel: w277 -> [w283 _]
              tunnel: w274 -> [w282 _]
              frame True {
                n82 = invoke class="VI" method="FP.Open"(reference=w283, error in=w284, "State"=w282) -> (error out=w285:errorcluster)  [unwired: 2 in, 4 out]
              }
              frame False {
              }
            }
          }
          frame "Minimize", "Minimized" {
            w287 = T1."Minimized" ("State")
            n83 = property class="VI"(reference=w293, error in=w292) -> (reference out=w290:refnum<vi>, error out=w291:errorcluster, "FP.State"=w289:T1)
            n84 = Not Equal?(x=w289, y=w287) -> (x != y?=w288:bool)
            n85 = case shown="True" w288 {
              tunnel: [w298 w299] -> w294
              tunnel: w291 -> [w297 w299]
              tunnel: w290 -> [w296 _]
              tunnel: w287 -> [w295 _]
              frame True {
                n86 = invoke class="VI" method="FP.Open"(reference=w296, error in=w297, "State"=w295) -> (error out=w298:errorcluster)  [unwired: 2 in, 4 out]
              }
              frame False {
              }
            }
          }
          frame "Maximize", "Maximized" {
            w300 = T1."Maximized" ("State")
            n87 = property class="VI"(reference=w306, error in=w305) -> (reference out=w303:refnum<vi>, error out=w304:errorcluster, "FP.State"=w302:T1)
            n88 = Not Equal?(x=w302, y=w300) -> (x != y?=w301:bool)
            n89 = case shown="True" w301 {
              tunnel: [w311 w312] -> w307
              tunnel: w304 -> [w310 w312]
              tunnel: w303 -> [w309 _]
              tunnel: w300 -> [w308 _]
              frame True {
                n90 = invoke class="VI" method="FP.Open"(reference=w309, error in=w310, "State"=w308) -> (error out=w311:errorcluster)  [unwired: 2 in, 4 out]
              }
              frame False {
              }
            }
          }
        }
      }
      frame "---------- Macro ----------" {
        n91 = call <vilib>:"Add State(s) to Queue__JKI_lib_State_Machine.vi"("State(s) in (\"\")"=w318) -> ("States Out"=w317:string)  [unwired: 14 in]
      }
      frame "Macro: Initialize" {
        w321 = "Data: Initialize\nInitialize Core Data\nEvents: Register\nUI: Initialize\n//Disable Open front panel to make it running behind\n//UI: Front Panel State >> Open"  # Data: Initialize Initialize Core Data Events: Register UI: Initialize //Disable Open front panel to make it running behind //UI: Front Panel State >> Open
        # "#CSM-Example Step 8.2 Disable Open front panel to make it running behind"
        n92 = call <vilib>:"Add State(s) to Queue__JKI_lib_State_Machine.vi"("State(s) in Front (\"\")"=w321, "State(s) in (\"\")"=w325) -> ("States Out"=w324:string)  [unwired: 13 in]
      }
      frame "Macro: Exit" {
        n93 = Unbundle By Name(w334) -> ("Core.Close Panel on Exit?"=w333:bool)
        n94 = Select(t="UI: Front Panel State >> Close", s=w333, f="") -> (s? t:f=w330:string)
        n95 = call <vilib>:"Add State(s) to Queue__JKI_lib_State_Machine.vi"("State(s) in (\"\")"=w330, "State(s) at Back (\"\")"="Data: Cleanup\nEvents: Unregister\nExit") -> ("States Out"=w328:string)  [unwired: 13 in]
        n96 = call <vilib>:"Add State(s) to Queue__JKI_lib_State_Machine.vi"("State(s) in Front (\"\")"=w328, "State(s) in (\"\")"=w337) -> ("States Out"=w336:string)  [unwired: 13 in]
      }
      frame "---------- API ----------" {
      }
      frame "API: Start" {
        # "#CSM-Example Step 6.1"
        n97 = call "CSM - Broadcast Status Change.vi"("Status With Arguments"="Check Started" ("Status with Arguments"), "State Queue"=w348) -> ("Remaining States"=w344:string)  [unwired: 13 in]
      }
      frame "API: Stop" {
        # "#CSM-Example Step 6.2"
        n98 = call "CSM - Broadcast Status Change.vi"("Status With Arguments"="Check Stoppped" ("Status with Arguments"), "State Queue"=w355) -> ("Remaining States"=w351:string)  [unwired: 13 in]
      }
      frame "API: Set Level" {
        # "#CSM-Example Step 6.3"
        n99 = Fract/Exp String To Number(string=w358) -> (number=w357:dbl)  [unwired: 3 in, 1 out]
        n100 = local write "Level"(w357) -> ()
        n101 = Bundle By Name(cluster=w362, "Level"=w357) -> (w359:T5)
      }
      frame "API: Get Level" {
        # "#CSM-Example Step 6.4"
        n102 = Unbundle By Name(w367) -> ("Level"=w366:dbl)
        n103 = Format Into String(w366) -> (resulting string=w365:string)  [unwired: 3 in, 1 out]
      }
      frame "---------- DoSth ----------" {
        n104 = call <vilib>:"Add State(s) to Queue__JKI_lib_State_Machine.vi"("State(s) in (\"\")"=w377) -> ("States Out"=w376:string)  [unwired: 14 in]
      }
      frame "DoSth: Check If Greater than 0.5" {
        # "#CSM-Example Step 3.2"
        # "#CSM-Example Step 3.1"
        # "#CSM-Example Step 3. Core functionality"
        n105 = Unbundle By Name(w382) -> ("Level"=w381:dbl)
        n106 = Random Number (0-1)() -> (number: 0 to 1=w387:dbl)
        "Random" <- w387
        n107 = Greater?(x=w387, y=w381) -> (0:w384:bool)
        "publish status" <- w384
        n108 = Format Into String(w387) -> (resulting string=w385:string)  [unwired: 3 in, 1 out]
        n109 = call <vilib>:"Build State String with Arguments__JKI_lib_State_Machine.vi"("Arguments (\"\")"=w385, "State"="Status Changed") -> ("State with Arguments"=w379:string)  [unwired: 4 in]
        n110 = call <vilib>:"Add State(s) to Queue__JKI_lib_State_Machine.vi"("State(s) in (\"\")"="Another Status" ("State"), "State(s) at Back (\"\")"=w379) -> ("States Out"=w378:string)  [unwired: 13 in]
        n111 = call "CSM - Broadcast Status Change.vi"("Status With Arguments"=w378, "State Queue"=w391, "Broadcast? (T)"=w384) -> ("Remaining States"=w390:string)  [unwired: 12 in]
      }
    }
  }
